vi "mediaRobos_v2.vi"(9 "Lado":enum16{"Esquerdo", "Direito"}(ring) caption="Enum", 10 "Field Size 2":T2, 11 "Array Robot Pose + CamID":T1(array[cluster])) -> (3 "Array":cluster{"x":dbl, "y":dbl, "robot_id":i32}[](array[cluster]))   [LabVIEW 2018]
panel:
  in  "file path (use dialog) 2":path=path "C:/Users/RoboIme/git/sslview/Util/Farias2.csv"
  in  "cluster":cluster{"x":dbl, "y":dbl, "robot_id":i32}
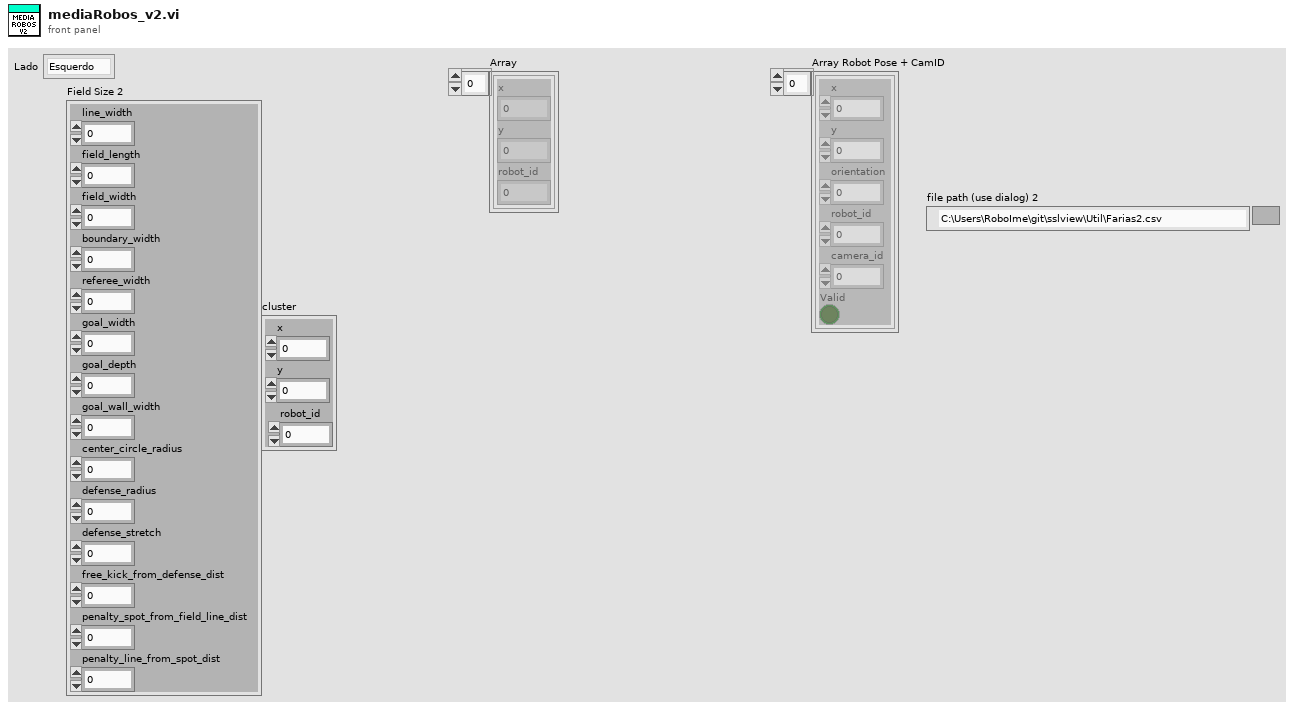
[diagram p1: front panel]
types:
  T1 = cluster{"x":sgl, "y":sgl, "orientation":sgl, "robot_id":u32, "camera_id":u32, "Valid":bool}[]
  T2 = cluster{"line_width":u32, "field_length":u32, "field_width":u32, "boundary_width":u32, "referee_width":u32, "goal_width":u32, "goal_depth":u32, "goal_wall_width":u32, "center_circle_radius":u32, "defense_radius":u32, "defense_stretch":u32, "free_kick_from_defense_dist":u32, "penalty_spot_from_field_line_dist":u32, "penalty_line_from_spot_dist":u32}
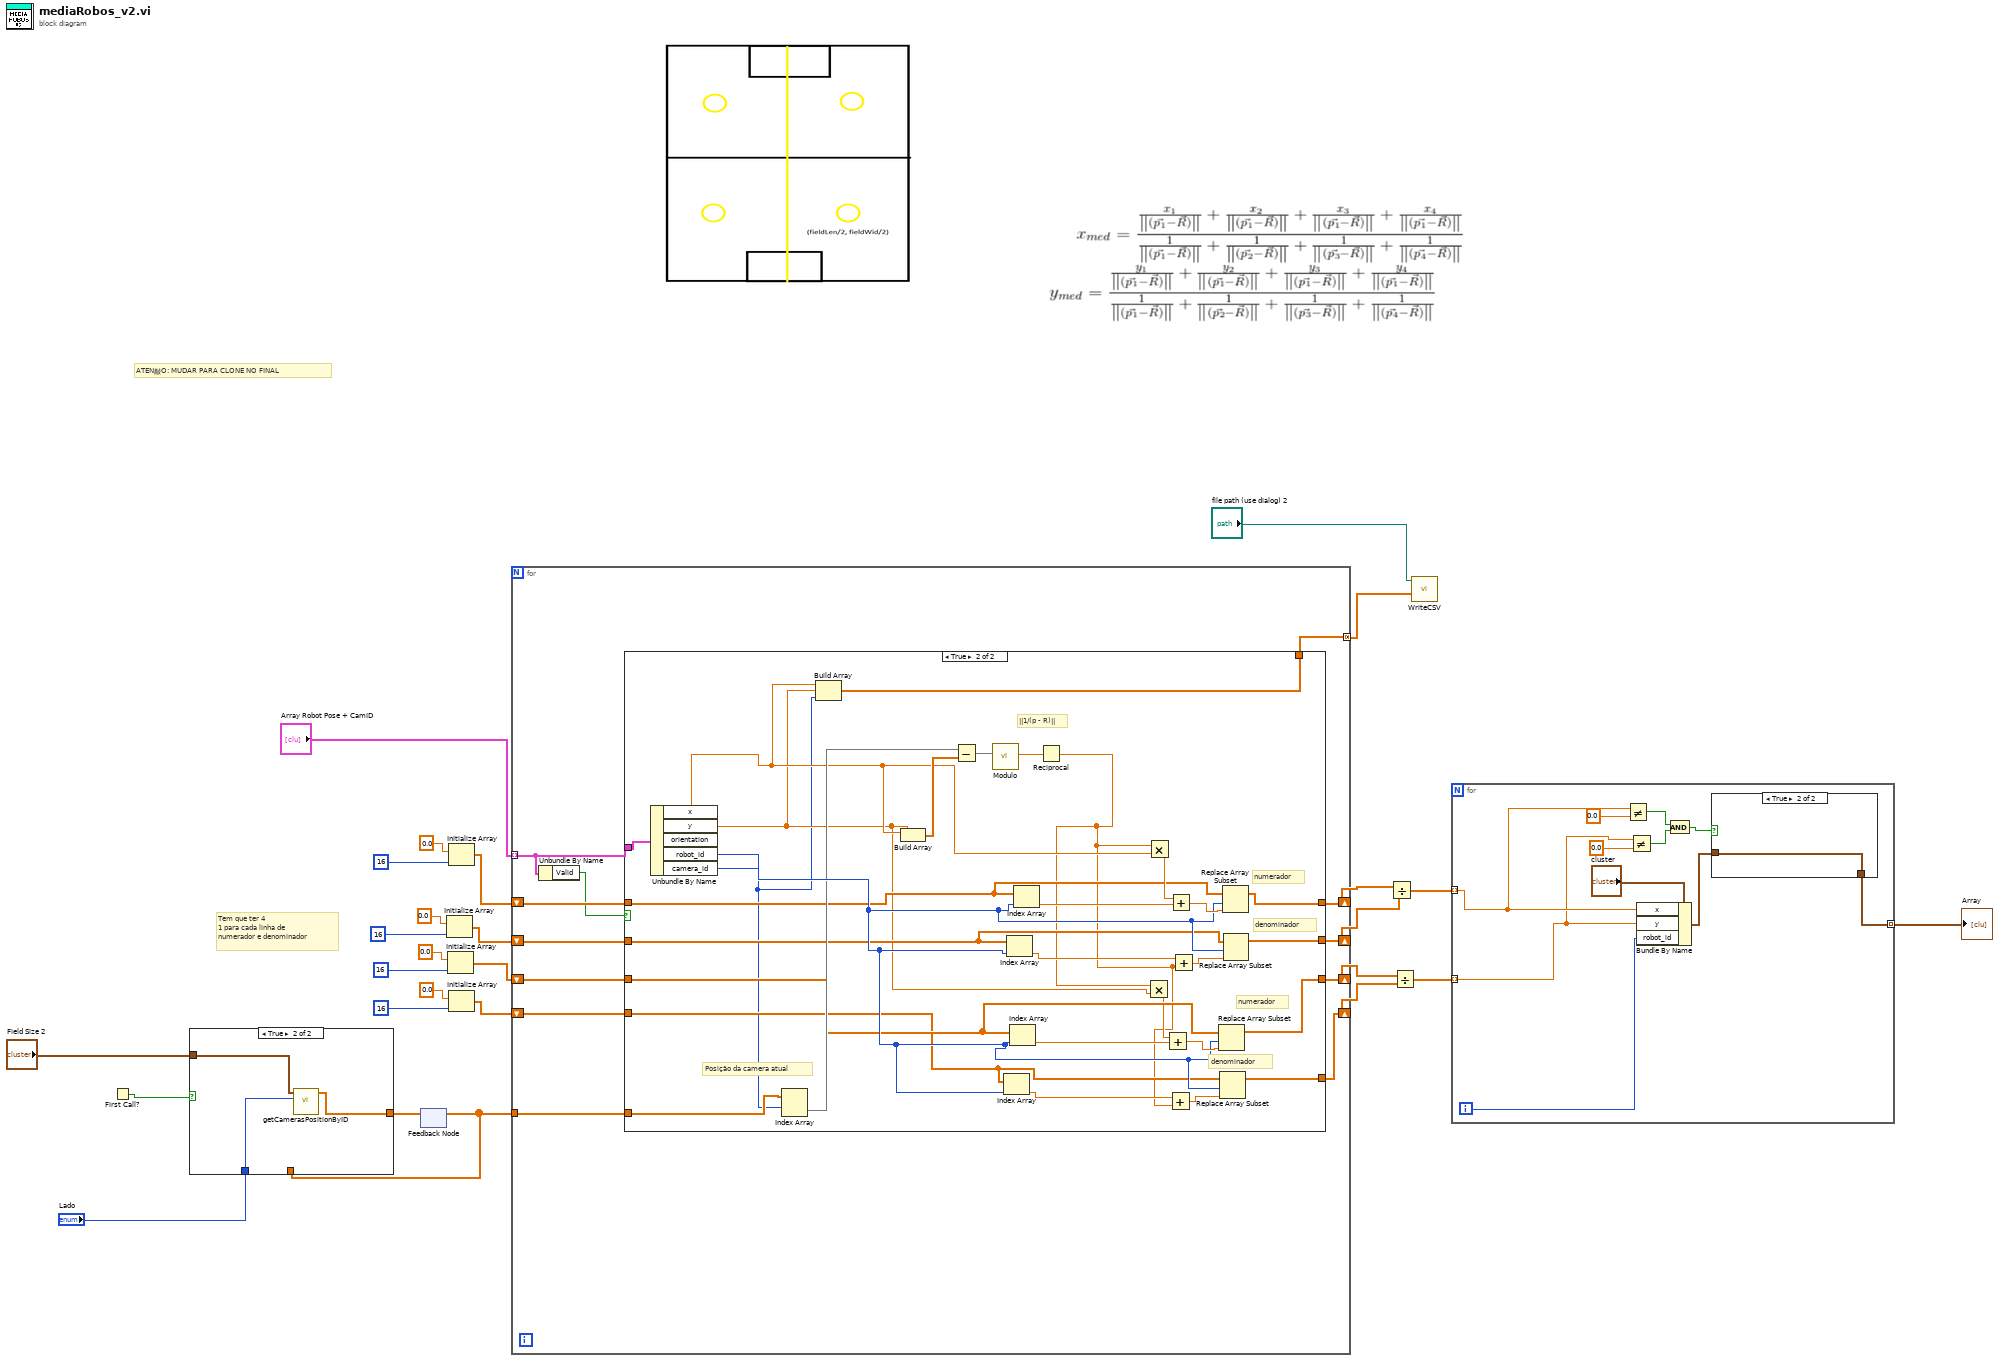
[diagram p0: block diagram]
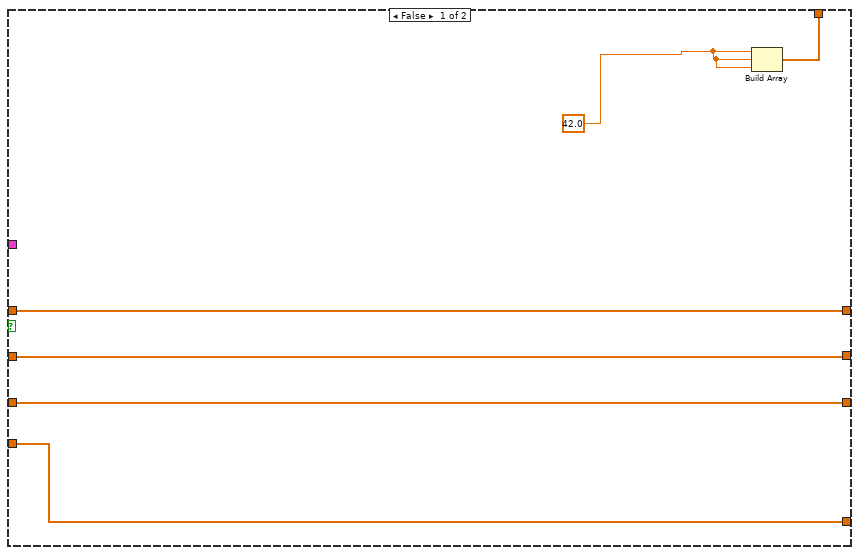
[diagram p4: hidden frame]
diagram:
  # "Tem que ter 4\n1 para cada linha de\nnumerador e denominador"
  # "ATEN敲O: MUDAR PARA CLONE NO FINAL"
  n1 = First Call?() -> (First Call?: T/F=w4:bool)
  n2 = feedback #1() -> (w2:dbl[][])  [unwired: 1 in]
  n3 = case shown="True" w4 {
    tunnel: "Field Size 2" -> [_ w31]
    tunnel: [w28 w30] -> w3
    tunnel: w2 -> [w28 _]
    tunnel: "Lado" -> [_ w29]
    frame False {
    }
    frame True {
      n4 = call "getCamerasPositionByID.vi"("Lado"=w29, "Field Size 2"=w31) -> ("Cameras Positions"=w30:dbl[][])  [unwired: 9 in]
    }
  }
  n5 = feedback-in #1(w3) -> ()
  n6 = Initialize Array(0.0 ("element"), 16 ("dimension size")) -> (w18:dbl[])
  n7 = Initialize Array(0.0 ("element"), 16 ("dimension size")) -> (w17:dbl[])
  n8 = Initialize Array(0.0 ("element"), 16 ("dimension size")) -> (w19:dbl[])
  n9 = Initialize Array(0.0 ("element"), 16 ("dimension size")) -> (w16:dbl[])
  n10 = for {
    tunnel: "Array Robot Pose + CamID" -> [w33] mode=indexing
    tunnel: w2 -> [w43]
    shift-right: [w42] -> w15
    shift-left: w19 -> [w36]
    shift-right: [w41] -> w14
    shift-left: w18 -> [w35]
    shift-right: [w40] -> w13
    shift-left: w17 -> [w38]
    shift-right: [w39] -> w12
    shift-left: w16 -> [w37]
    tunnel: [w34] -> w7 mode=concatenating
    n11 = Unbundle By Name(w33) -> ("Valid"=w32:bool)
    n12 = case shown="True" w32 {
      tunnel: w33 -> [_ w79]
      tunnel: w43 -> [_ w78]
      tunnel: [w49 w63] -> w42
      tunnel: [w48 w62] -> w41
      tunnel: [w47 w61] -> w40
      tunnel: [w46 w60] -> w39
      tunnel: w38 -> [w47 w59]
      tunnel: w37 -> [w46 w58]
      tunnel: w36 -> [w49 w57]
      tunnel: w35 -> [w48 w56]
      tunnel: [w45 w51] -> w34
      frame False {
        w44 = 42.0 ("element")
        n13 = Build Array(w44, w44, w44) -> (w45:dbl[])
      }
      frame True {
        # "denominador"
        # "numerador"
        # "denominador"
        # "numerador"
        # "||1/(p - R)||"
        # "Posição da camera atual"
        n14 = Unbundle By Name(w79) -> ("x"=w54:sgl, "y"=w53:sgl, "robot_id"=w69:u32, "camera_id"=w52:u32)  [unwired: 1 out]
        n15 = Index Array(array=w78, index (row)=w52) -> (element=w68:dbl[])  [unwired: 1 in]
        n16 = Build Array(w54, w53, w52) -> (w51:sgl[])
        n17 = Build Array(w54, w53) -> (w77:sgl[])
        n18 = Subtract(x=w68, y=w77) -> (x-y=w76:dbl[])
        n19 = call "Modulo.vi"("2D vector"=w76) -> ("Modulo"=w75:dbl)  [unwired: 10 in]
        n20 = Index Array(array=w58, index=w69) -> (element=w64:dbl)
        n21 = Index Array(array=w56, index=w69) -> (element=w66:dbl)
        n22 = Index Array(array=w59, index=w69) -> (element=w65:dbl)
        n23 = Index Array(array=w57, index=w69) -> (element=w67:dbl)
        n24 = Reciprocal(x=w75) -> (1/x=w50:dbl)
        n25 = Multiply(x=w50, y=w53) -> (x*y=w55:dbl)
        n26 = Multiply(x=w50, y=w54) -> (x*y=w74:dbl)
        n27 = Add(x=w55, y=w65) -> (x+y=w71:dbl)
        n28 = Add(x=w64, y=w50) -> (x+y=w70:dbl)
        n29 = Add(x=w74, y=w67) -> (x+y=w73:dbl)
        n30 = Add(x=w66, y=w50) -> (x+y=w72:dbl)
        n31 = Replace Array Subset(array=w59, new element=w71, index=w69) -> (w61:dbl[])
        n32 = Replace Array Subset(array=w58, new element=w70, index=w69) -> (w60:dbl[])
        n33 = Replace Array Subset(array=w57, new element=w73, index=w69) -> (w63:dbl[])
        n34 = Replace Array Subset(array=w56, new element=w72, index=w69) -> (w62:dbl[])
      }
    }
  }
  n35 = Divide(x=w15, y=w14) -> (x/y=w11:dbl[])
  n36 = Divide(x=w13, y=w12) -> (x/y=w10:dbl[])
  n37 = call "WriteCSV.vi"("array"=w7, "file path (use dialog)"="file path (use dialog) 2") -> ()  [unwired: 10 in]
  n38 = for {
    tunnel: w11 -> [w89] mode=indexing
    tunnel: w10 -> [w86] mode=indexing
    tunnel: [w82] -> w9 mode=indexing
    i -> [w90]
    n39 = Not Equal?(x=w89, y=0.0) -> (x != y?=w85:bool)
    n40 = Not Equal?(x=w86, y=0.0) -> (x != y?=w84:bool)
    n41 = Bundle By Name(cluster="cluster", "x"=w89, "y"=w86, "robot_id"=w90) -> (w81:cluster{"x":dbl, "y":dbl, "robot_id":i32})
    n42 = And(x=w85, y=w84) -> (x .and. y?=w83:bool)
    n43 = case shown="True" w83 {
      tunnel: [w91 w92] -> w82
      tunnel: w81 -> [w91 w92]
      frame False {
      }
      frame True {
      }
    }
  }
  "Array" <- w9
